vi "Log Data.vi"(8 "error in (no error)":errorcluster, 11 "Sensor & Control in":refnum<class "Sensor & Control.lvclass">) -> (0 "error out":errorcluster, 3 "Sensor & Control out":refnum<class "Sensor & Control.lvclass">)   [LabVIEW 2013, in "Sensor & Control.lvib.lvlib" / "Sensor & Control.lvclass"]
uses:
  Sensor & Control.lvclass
  Sensor & Control.lvclass/Sensor & Control.ctl
  Read Value.vi
  Read Setpoint.vi
  PluginInterface/PluginInterface.lvlibp/PluginInterfaceClass/Read TDMS.vi
  PluginInterface/PluginInterface.lvlibp/PluginInterfaceClass/Read Name.vi
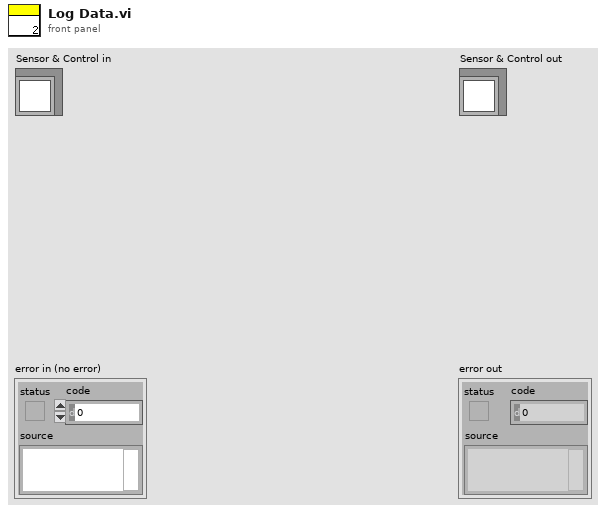
[diagram p1: front panel]
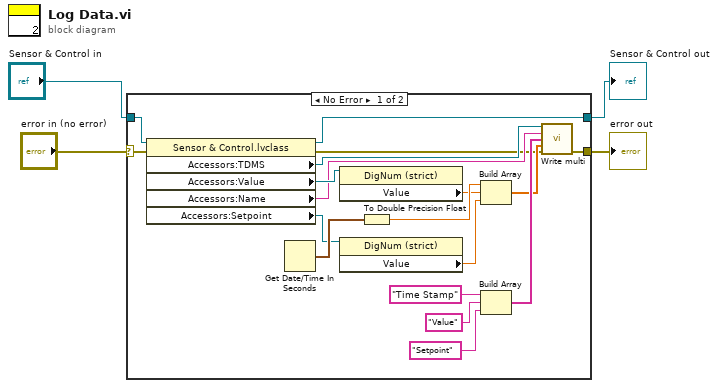
[diagram p0: block diagram]
diagram:
  n1 = case shown="No Error" "error in (no error)" {
    selector: "error in (no error)" -> [w14 w24]
    tunnel: [w13 w24] -> w3
    tunnel: [w5 w23] -> w1
    tunnel: "Sensor & Control in" -> [w21 w23]
    frame No Error {
      n2 = property class="Sensor & Control.lvclass"(reference=w21, error in=w14) -> (reference out=w5:refnum<class "Sensor & Control.lvclass">, error out=w6:errorcluster, "Accessors:TDMS"=w20:refnum<k34>, "Accessors:Value"=w12:refnum<vi>, "Accessors:Name"=w7:string, "Accessors:Setpoint"=w11:refnum<vi>)
      n3 = Get Date/Time In Seconds() -> (seconds since 1Jan1904=w22:timestamp)
      n4 = property class="DigNum (strict)"(reference=w12) -> ("Value"=w10:dbl)  [unwired: 1 in, 2 out]
      n5 = property class="DigNum (strict)"(reference=w11) -> ("Value"=w9:dbl)  [unwired: 1 in, 2 out]
      n6 = To Double Precision Float(number=w22) -> (double precision float=w15:dbl)
      n7 = Build Array(w15, w10, w9) -> (w8:dbl[])
      n8 = Build Array("Time Stamp" ("Channel"), "Value" ("string"), "Setpoint" ("string")) -> (w16:string[])
      n9 = call "Write multi.vi"("tdms file in"=w20, "group"=w7, "Channel"=w16, "Data"=w8, "error in (no error)"=w6) -> ("error out"=w13:errorcluster)  [unwired: 7 in, 3 out]
    }
    frame Error {
    }
  }
  "error out" <- w3
  "Sensor & Control out" <- w1
